vi "Find Goals.vi"(9 "Color":T1, 10 "Image Dst":T2, 11 "Image Src":T2) -> ()   [LabVIEW 2015]
uses:
  <vilib>/vision/Image Controls.llb/IMAQ Image.ctl
  <vilib>/vision/NI_Vision_Development_Module.lvlib
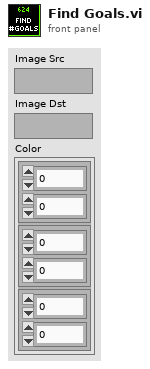
[diagram p1: front panel]
types:
  T1 = cluster{cluster{dbl, dbl}, cluster{dbl, dbl}, cluster{dbl, dbl}}
  T2 = typedef "IMAQ Image.ctl" = refnum<image>
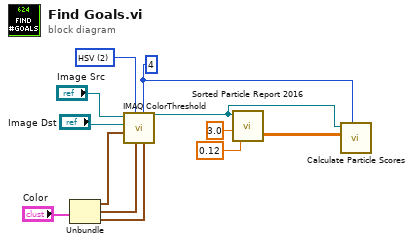
[diagram p0: block diagram]
diagram:
  w1 = 4 ("Replace Value")
  w10 = u16 2 items=["RGB", "HSL", "HSV", "HSI"] ("Color Mode")
  n1 = Unbundle("Color") -> (w8:cluster{dbl, dbl}, w7:cluster{dbl, dbl}, w6:cluster{dbl, dbl})
  n2 = call "IMAQ ColorThreshold"("Blue or Luma or Val or Inten Range"=w6, "Replace Value"=w1, "Green or Sat Range"=w7, "Color Mode"=w10, "Red or Hue Range"=w8, "Image Dst"="Image Dst", "Image Src"="Image Src") -> ("Image Dst Out"=w2:T2)  [unwired: 3 in, 1 out]
  n3 = call "Sorted Particle Report 2016.vi"("Min Area Size %"=0.12, "Particle Count Limit"=3.0, "Image in"=w2) -> ("Sorted Data"=w3:dbl[][])  [unwired: 1 in, 1 out]
  n4 = call "Calculate Particle Scores.vi"("Pixel Value"=w1, "Sorted Data"=w3, "Image in"=w2) -> ()  [unwired: 8 in, 1 out]
